vi "outgoing data.vi"(6 "timeout (-1)":i32=-1, 8 "error in":errorcluster, 11 "websocket user plugin in":refnum<class "websocket user plugin.lvclass">) -> (0 "error out":errorcluster, 1 "timeout":bool, 2 "opcode":u8=1, 3 "data":string, 5 "not last fragment (F)":bool, 7 "kill connection":bool)   [LabVIEW 2016, in "websocket user plugin.lvclass"]
uses:
  websocket user plugin.lvclass
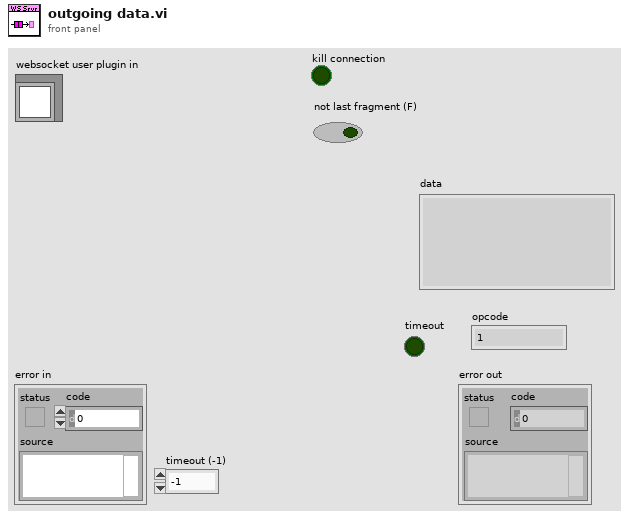
[diagram p1: front panel]
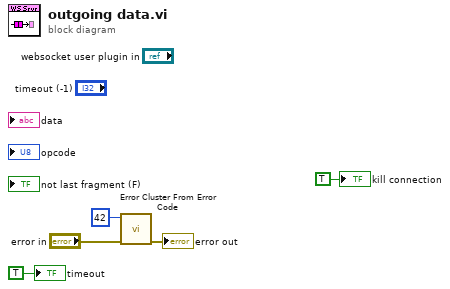
[diagram p0: block diagram]
diagram:
  n1 = call <vilib>:"Error Cluster From Error Code.vi"("error in (no error)"="error in", "error code (0)"=42) -> ("error out"=→"error out":errorcluster)  [unwired: 7 in]
  "timeout" <- TRUE ("timeout")
  "kill connection" <- TRUE
